vi "AlliGator Calibrated Phasor Map Series Dialog.vi"(5 "error in (no error)":errorcluster) -> (13 "OK":bool, 15 "Calibration Map/Gate Step List":T1[](array[typedef]), 16 "Destination Folder":path, 17 "File Suffix (# Steps will be added)":string caption="File Name (# Steps will be added)", 18 "Save Phasor Plot":bool caption="Save Phasor Map", 19 "error out":errorcluster)   [LabVIEW 2021, in "AlliGator Scripts.lvlib"]
doc: "Dialog window to enter the information eeded to run the Calibrated Phasor Map Series script."
uses:
  AlliGator Scripts.lvlib
  AlliGator Dataset + Calibration Map + Gate Step.ctl
panel:
  in  "Save Phasor Plot":bool
  in  "Dataset/Calibration Map/Gate Step List":T1[](array[typedef]) caption="Dataset/Calibration Map/Gate Step List:"
  in  "File Suffix (# Steps will be added)":string caption="File Name (# Steps will be added)"
  in  "Destination Folder":path
  in  "Cancel":bool
  in  "OK2":bool
  # "Enter the information needed to compute the series\nof calibrated phasor plots for each dataset:"
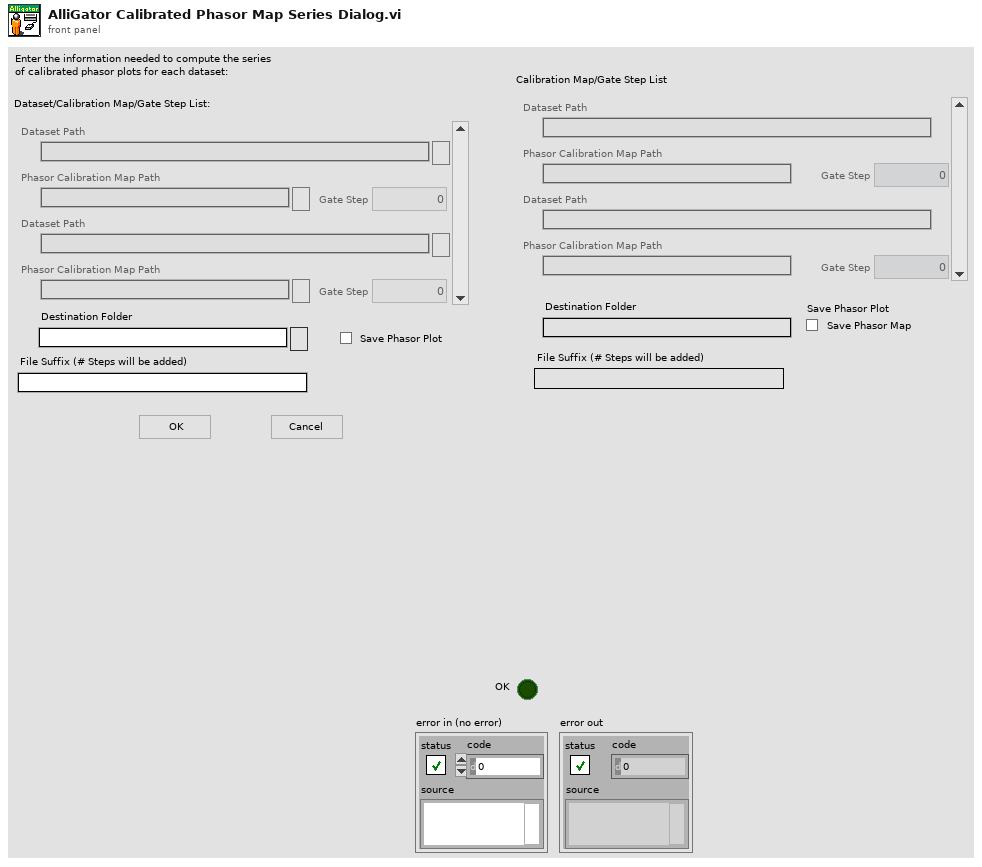
[diagram p1: front panel]
types:
  T1 = typedef "AlliGator Scripts.lvlib/AlliGator Dataset + Calibration Map + Gate Step.ctl" = cluster{"Phasor Calibration Map Path":path, "Gate Step":i32, "Dataset Path":path}
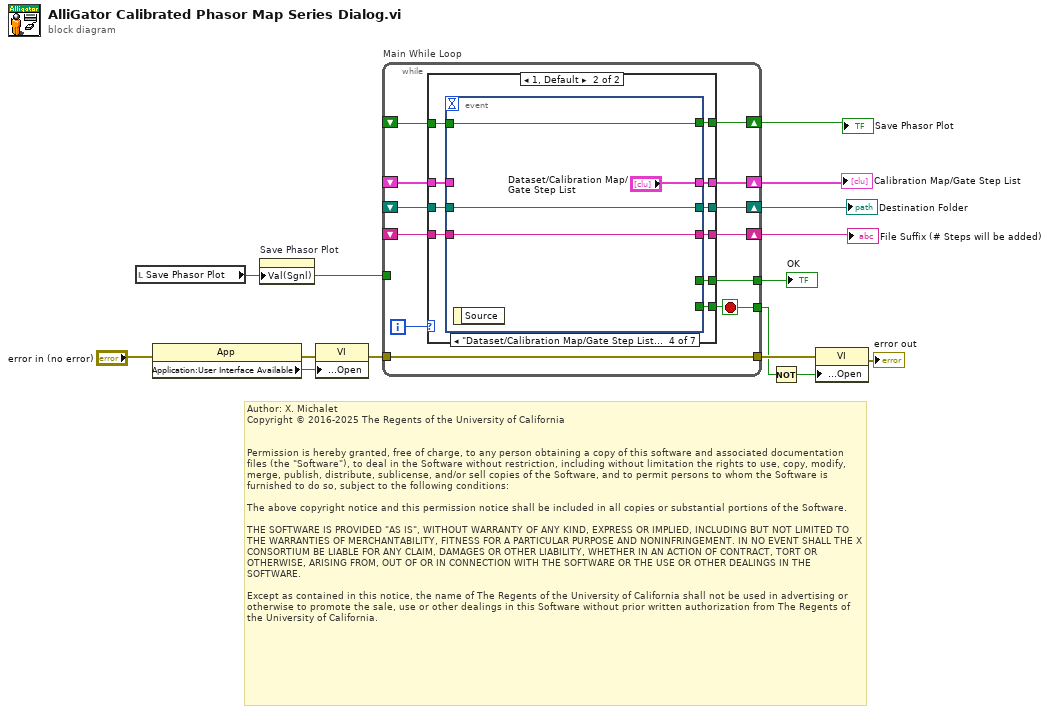
[diagram p0: block diagram]
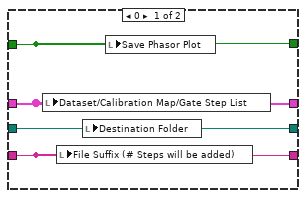
[diagram p2: hidden frame]
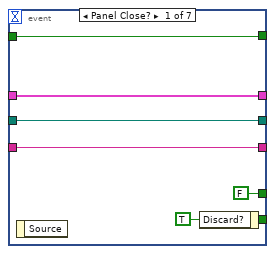
[diagram p3: hidden frame]
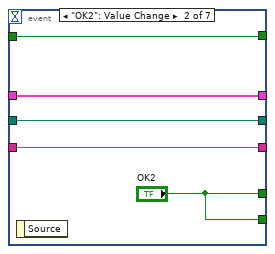
[diagram p4: hidden frame]
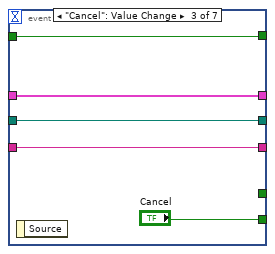
[diagram p5: hidden frame]
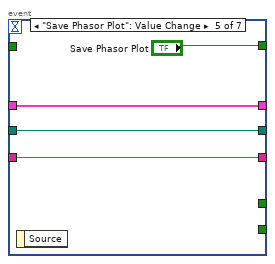
[diagram p6: hidden frame]
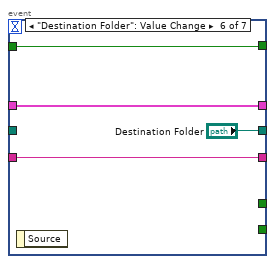
[diagram p7: hidden frame]
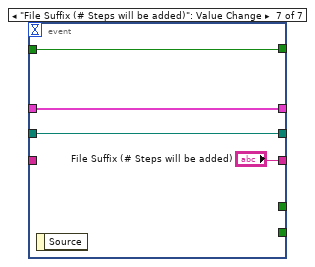
[diagram p8: hidden frame]
diagram:
  # "Author: X. Michalet\nCopyright © 2016-2025 The Regents of the University of California\n \n\nPermission is hereby granted, free of charge, to any person obtaining a copy of this software and associated documentation files (the \"Software\"), to deal in the Software without restriction, including without limitation the rights to use, copy, modify, merge, publish, distribute, sublicense, and/or sell copies of the Software, and to permit persons to whom the Software is furnished to do so, subject to the following conditions:\n\nThe above copyright notice and this permission notice shall be included in all copies or substantial portions of the Software.\n\nTHE SOFTWARE IS PROVIDED \"AS IS\", WITHOUT WARRANTY OF ANY KIND, EXPRESS OR IMPLIED, INCLUDING BUT NOT LIMITED TO THE WARRANTIES OF MERCHANTABILITY, FITNESS FOR A PARTICULAR PURPOSE AND NONINFRINGEMENT. IN NO EVENT SHALL THE X CONSORTIUM BE LIABLE FOR ANY CLAIM, DAMAGES OR OTHER LIABILITY, WHETHER IN AN ACTION OF CONTRACT, TORT OR OTHERWISE, ARISING FROM, OUT OF OR IN CONNECTION WITH THE SOFTWARE OR THE USE OR OTHER DEALINGS IN THE SOFTWARE.\n\nExcept as contained in this notice, the name of The Regents of the University of California shall not be used in advertising or otherwise to promote the sale, use or other dealings in this Software without prior written authorization from The Regents of the University of California."
  n1 = local read "Save Phasor Plot"() -> (w1:bool)
  n2 = property class="App"(error in="error in (no error)") -> (error out=w9:errorcluster, "Application:User Interface Available"=w11:bool)  [unwired: 1 in, 1 out]
  n3 = property on="Save Phasor Plot" class="Bool (strict)"("Val(Sgnl)"=w1) -> ()  [unwired: 2 in, 2 out]
  n4 = property class="VI"(error in=w9, "Front Panel Window:Open"=w11) -> (error out=w14:errorcluster)  [unwired: 1 in, 1 out]
  n5 = while "Main While Loop" {
    tunnel: w14 -> [w26]
    tunnel: [w26] -> w13
    tunnel: [w25] -> w8
    tunnel: [w24] -> w7
    shift-right: [w23] -> w2
    shift-left: _ -> [w21]
    shift-right: [w22] -> w5
    shift-left: _ -> [w19]
    shift-right: [w20] -> w4
    shift-left: _ -> [w18]
    shift-right: [w16] -> w3
    shift-left: _ -> [w15]
    tunnel: w1 -> [_]
    i -> [w17]
    stop <- w24 stop-if-true
    n6 = case shown="1, Default" w17 {
      tunnel: [_ w40] -> w25
      tunnel: [_ w39] -> w24
      tunnel: [w30 w38] -> w23
      tunnel: [w28 w37] -> w22
      tunnel: w21 -> [w30 w36]
      tunnel: [w29 w35] -> w20
      tunnel: w19 -> [w28 w34]
      tunnel: w18 -> [w29 w33]
      tunnel: [w27 w32] -> w16
      tunnel: w15 -> [w27 w31]
      frame 0 {
        n7 = local write "Dataset/Calibration Map/Gate Step List"(w30) -> ()
        n8 = local write "File Suffix (# Steps will be added)"(w29) -> ()
        n9 = local write "Destination Folder"(w28) -> ()
        n10 = local write "Save Phasor Plot"(w27) -> ()
      }
      frame 1, Default {
        n11 = event shown="[3] \"Dataset/Calibration Map/Gate Step List\": Value Change" {
          selector: _ -> [_ _ _ _ _ _ _]
          dyn-events: _ -> [_ _ _ _ _ _ _]
          timeout: _ -> [_ _ _ _ _ _ _]
          tunnel: [w46 "OK2" "Cancel" _ _ _ _] -> w39
          tunnel: [FALSE ("OK") "OK2" _ _ _ _ _] -> w40
          tunnel: [w44 w50 w55 "Dataset/Calibration Map/Gate Step List" w62 w67 w72] -> w38
          tunnel: [w43 w49 w54 w60 w64 "Destination Folder" w70] -> w37
          tunnel: w36 -> [w44 w50 w55 _ w62 w67 w72]
          tunnel: [w42 w48 w53 w59 w63 w66 "File Suffix (# Steps will be added)"] -> w35
          tunnel: w34 -> [w43 w49 w54 w60 w64 _ w70]
          tunnel: w33 -> [w42 w48 w53 w59 w63 w66 _]
          tunnel: [w41 w47 w52 w57 "Save Phasor Plot" w65 w69] -> w32
          tunnel: w31 -> [w41 w47 w52 w57 _ w65 w69]
          event Panel Close? {
            w46 = TRUE ("Discard?")
            n12 = event-data() -> ()  [unwired: 1 in, 1 out]
            n13 = event-data("Discard?"=w46) -> ()  [unwired: 1 in, 1 out]
          }
          event "OK2": Value Change {
            n14 = event-data() -> ()  [unwired: 1 in, 1 out]
          }
          event "Cancel": Value Change {
            n15 = event-data() -> ()  [unwired: 1 in, 1 out]
          }
          event "Dataset/Calibration Map/Gate Step List": Value Change {
            n16 = event-data() -> ()  [unwired: 1 in, 1 out]
          }
          event "Save Phasor Plot": Value Change {
            n17 = event-data() -> ()  [unwired: 1 in, 1 out]
          }
          event "Destination Folder": Value Change {
            n18 = event-data() -> ()  [unwired: 1 in, 1 out]
          }
          event "File Suffix (# Steps will be added)": Value Change {
            n19 = event-data() -> ()  [unwired: 1 in, 1 out]
          }
        }
      }
    }
  }
  "OK" <- w8
  "Destination Folder" <- w5
  "File Suffix (# Steps will be added)" <- w4
  "Calibration Map/Gate Step List" <- w2
  "Save Phasor Plot" <- w3
  n20 = Not(x=w7) -> (.not. x?=w6:bool)
  n21 = property class="VI"(error in=w13, "Front Panel Window:Open"=w6) -> (error out=→"error out":errorcluster)  [unwired: 1 in, 1 out]
